vi "SettingsEngine.vi"(7 "Enum":T1, 8 "error in":errorcluster, 10 "New Setting Value":string, 11 "Setting Name":string) -> (0 "error out":errorcluster, 2 "Setting Value":string)   [LabVIEW 2009]
uses:
  SettingsEngineEnum.ctl
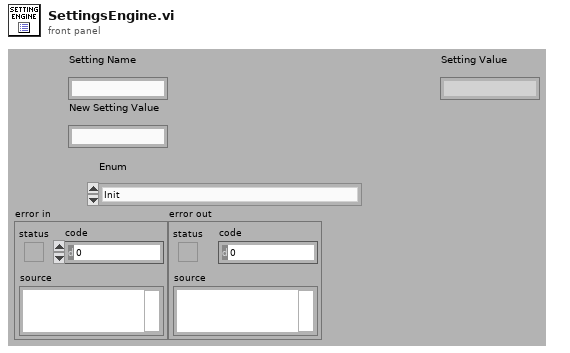
[diagram p1: front panel]
types:
  T1 = typedef "SettingsEngineEnum.ctl" = enum16{"Init", "Load Settings from File", "Get Setting", "Set/Create Setting", "Save Settings to File"}
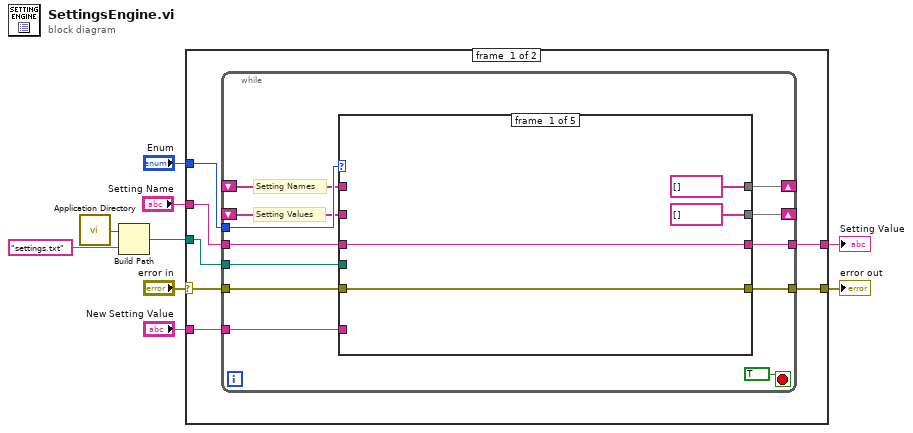
[diagram p0: block diagram]
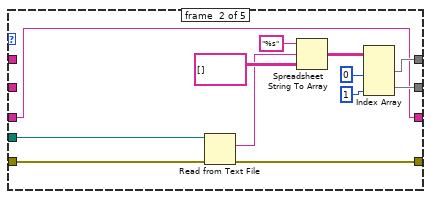
[diagram p2: hidden frame]
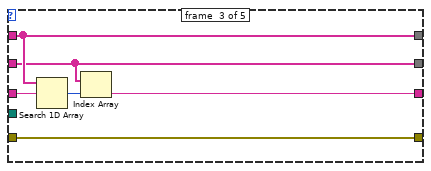
[diagram p3: hidden frame]
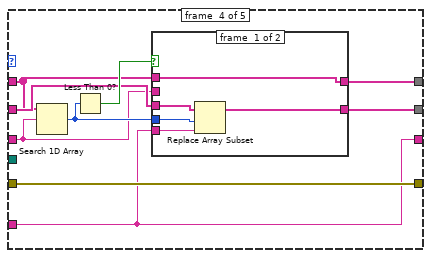
[diagram p4: hidden frame]
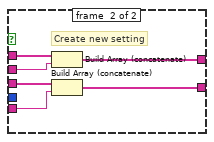
[diagram p5: hidden frame]
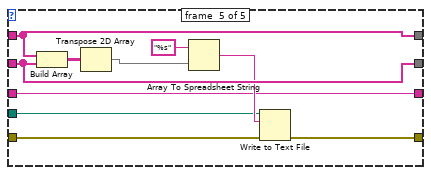
[diagram p6: hidden frame]
diagram:
  n1 = call <vilib>:"Application Directory.vi"() -> ("Application Directory"=w5:path)
  n2 = Build Path(base path=w5, name or relative path="settings.txt") -> (appended path=w4:path)
  n3 = case shown="No Error" "error in" {
    selector: "error in" -> [w15 w82]
    tunnel: "Enum" -> [w16 _]
    tunnel: [w14 w82] -> w7
    tunnel: w4 -> [w13 _]
    tunnel: "Setting Name" -> [w12 w81]
    tunnel: [w11 w81] -> w2
    tunnel: "New Setting Value" -> [w10 _]
    frame #0 {
      n4 = while {
        tunnel: w16 -> [w27]
        shift-right: [w26] -> _
        shift-left: _ -> [w25]
        shift-right: [w24] -> _
        shift-left: _ -> [w23]
        tunnel: w15 -> [w22]
        tunnel: [w21] -> w14
        tunnel: w13 -> [w20]
        tunnel: w12 -> [w19]
        tunnel: [w18] -> w11
        tunnel: w10 -> [w17]
        stop <- TRUE ("stop") stop-if-true
        # "Setting Values"
        # "Setting Names"
        n5 = case shown="\"Save Settings to File\"" w27 {
          tunnel: [string[] [] w36 w49 w53 w80] -> w26
          tunnel: w25 -> [_ _ w49 w52 w80]
          tunnel: [string[] [] w35 w47 w54 w79] -> w24
          tunnel: w23 -> [_ _ w47 w57 w79]
          tunnel: w22 -> [w30 w44 w50 w59 w73]
          tunnel: [w30 w43 w50 w59 w72] -> w21
          tunnel: w20 -> [_ w34 _ _ w74]
          tunnel: w19 -> [w29 w33 w48 w51 w71]
          tunnel: [w29 w33 w45 w56 w71] -> w18
          tunnel: w17 -> [_ _ _ w56 _]
          frame #0 {
          }
          frame #1 {
            n6 = Read from Text File(file (use dialog)=w34, error in=w44) -> (text=w41:string, error out=w43:errorcluster)  [unwired: 2 in, 2 out]
            n7 = Spreadsheet String To Array(format string="%s", spreadsheet string=w41, array type (2D Dbl)=string[][] []) -> (array=w39:string[][])  [unwired: 1 in]
            n8 = Index Array(array=w39, index (col) #1=0 ("disabled index (col)"), index (col) #2=1 ("index (col)")) -> (element #1=w36:string[], element #2=w35:string[])  [unwired: 2 in]
          }
          frame #2 {
            n9 = Search 1D Array(1D array=w49, element=w48) -> (index of element=w46:i32)  [unwired: 1 in]
            n10 = Index Array(array=w47, index=w46) -> (element=w45:string)
          }
          frame #3 {
            n11 = Search 1D Array(1D array=w52, element=w51) -> (index of element=w55:i32)  [unwired: 1 in]
            n12 = Less Than 0?(x=w55) -> (x < 0?=w58:bool)
            n13 = case shown="True" w58 {
              tunnel: w57 -> [w64 w68]
              tunnel: w56 -> [w63 w65]
              tunnel: w55 -> [w62 _]
              tunnel: [w61 w67] -> w54
              tunnel: [w60 w69] -> w53
              tunnel: w52 -> [w60 w70]
              tunnel: w51 -> [_ w66]
              frame #0 {
                n14 = Replace Array Subset(array=w64, new element=w63, index=w62) -> (w61:string[])
              }
              frame #1 {
                # "Create new setting"
                n15 = Build Array (concatenate)(w70, w66) -> (w69:string[])
                n16 = Build Array (concatenate)(w68, w65) -> (w67:string[])
              }
            }
          }
          frame #4 {
            n17 = Build Array(w80, w79) -> (w77:string[][])
            n18 = Transpose 2D Array(2D array=w77) -> (transposed array=w76:string[][])
            n19 = Array To Spreadsheet String(array=w76, 3:"%s" ("format string")) -> (spreadsheet string=w75:string)  [unwired: 1 in]
            n20 = Write to Text File(file (use dialog)=w74, text=w75, error in=w73) -> (error out=w72:errorcluster)  [unwired: 1 in, 2 out]
          }
        }
      }
    }
    frame #1 {
    }
  }
  "error out" <- w7
  "Setting Value" <- w2
